vi "Choose_best_target(multi).vi"(0 "R1mag lower limit":dbl, 2 "FOV":dbl, 3 "Footprint":dbl, 5 "PM limit":dbl, 6 "EPOCH TEL":dbl format="%.3f", 8 "DEC TEL":dbl format="%<%H:%M:%S>t", 9 "Table Astrometry":T1 {"CRVAL" format="%.6g"; "CD" format="%_8g"; "NAXIS" format="%#.0f"}, 10 "RA TEL":dbl format="%<%H:%M:%S%1u>t", 12 "USNO_data":string[][](array[string])) -> (11 "Best Target":string[][](array[string]), 13 "erreur":bool, 14 "target RA":dbl format="%<%H:%M:%S%2u>t", 15 "target DEC":dbl format="%<%H:%M:%S%1u>t", 16 "target EPOCH":dbl format="%.3f", 17 "target R1mag":dbl format="%.2f", 18 "target RA (deg)":dbl format="%#.6f", 19 "target DEC (deg)":dbl format="%#.6f")   [LabVIEW 2019]
panel:
  out "tmp_data":string[][](array[string])
  out "R-I":dbl
  out "B-R":dbl
  out "target X":dbl
  out "target Y":dbl
  out "Data OUT":string[][](array[string])
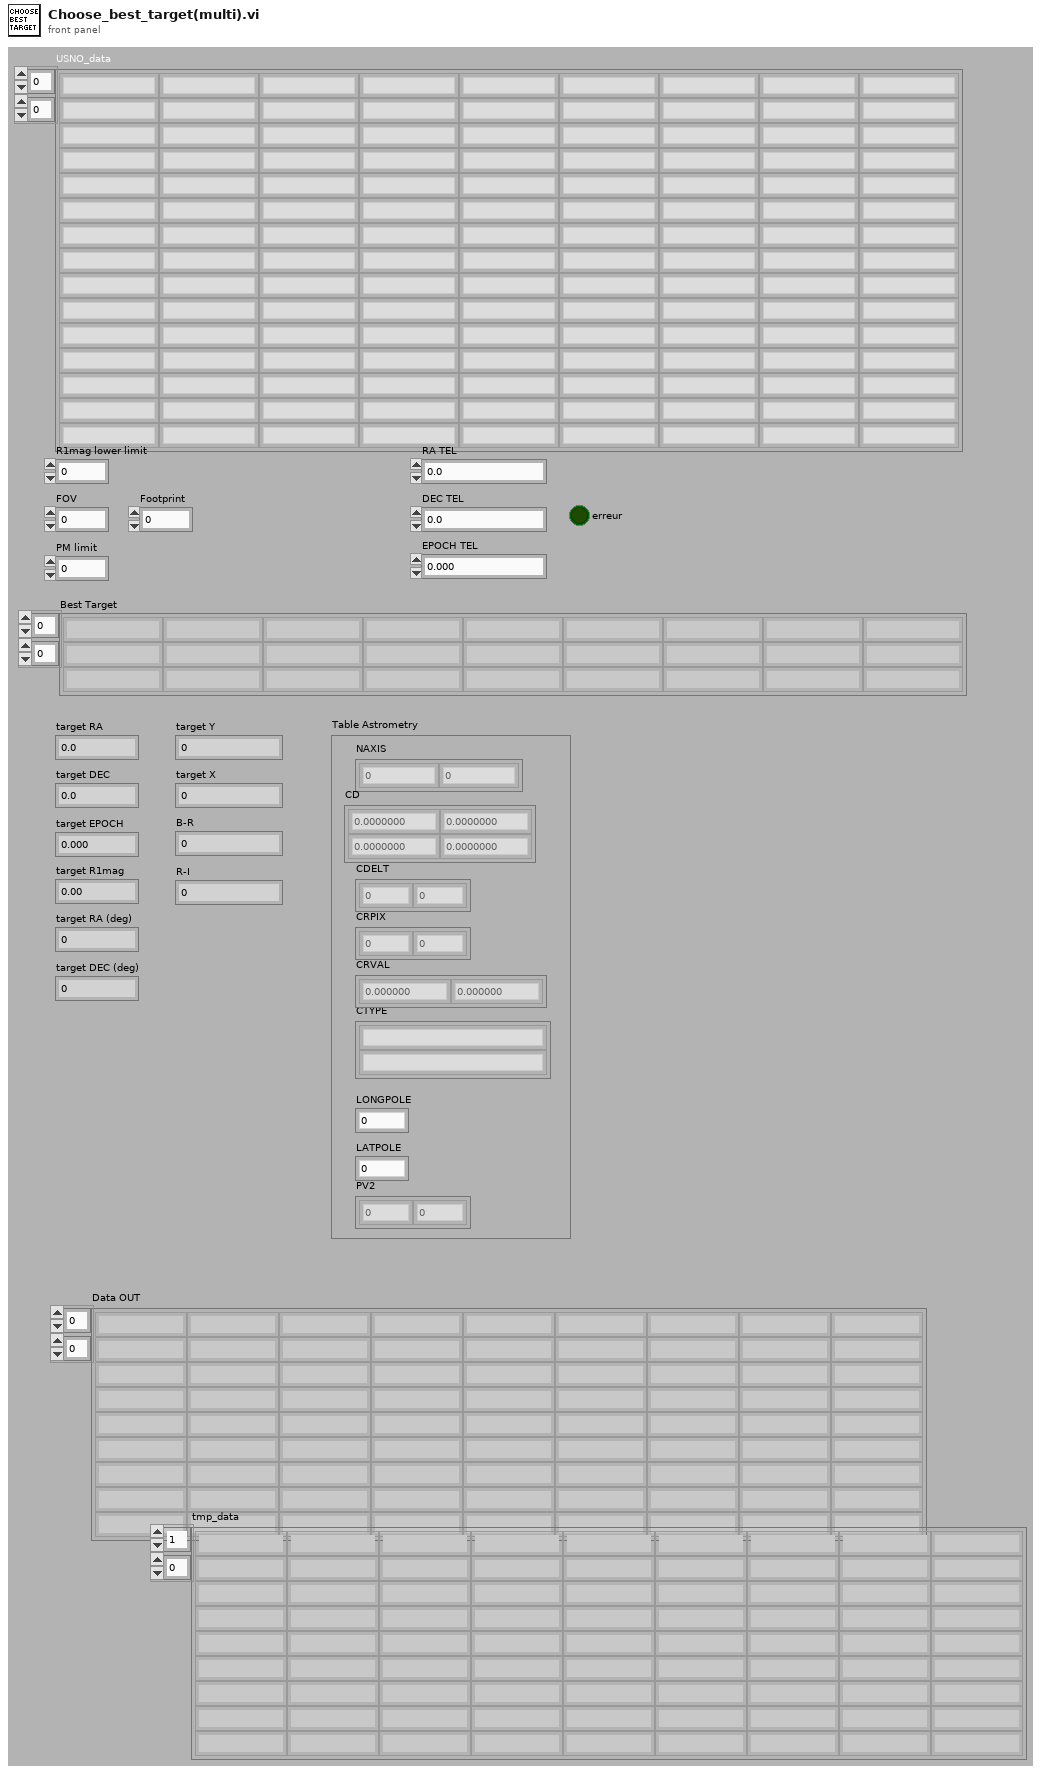
[diagram p1: front panel]
types:
  T1 = cluster{"NAXIS":dbl[], "CD":dbl[][], "CDELT":dbl[], "CRPIX":dbl[], "CTYPE":string[], "CRVAL":dbl[], "LONGPOLE":dbl, "LATPOLE":dbl, "PV2":dbl[]}
  T2 = cluster{"crit":string, "String":string, "String":string, "String":string, "String":string, "String":string, "String":string, "String":string, "String":string}[]
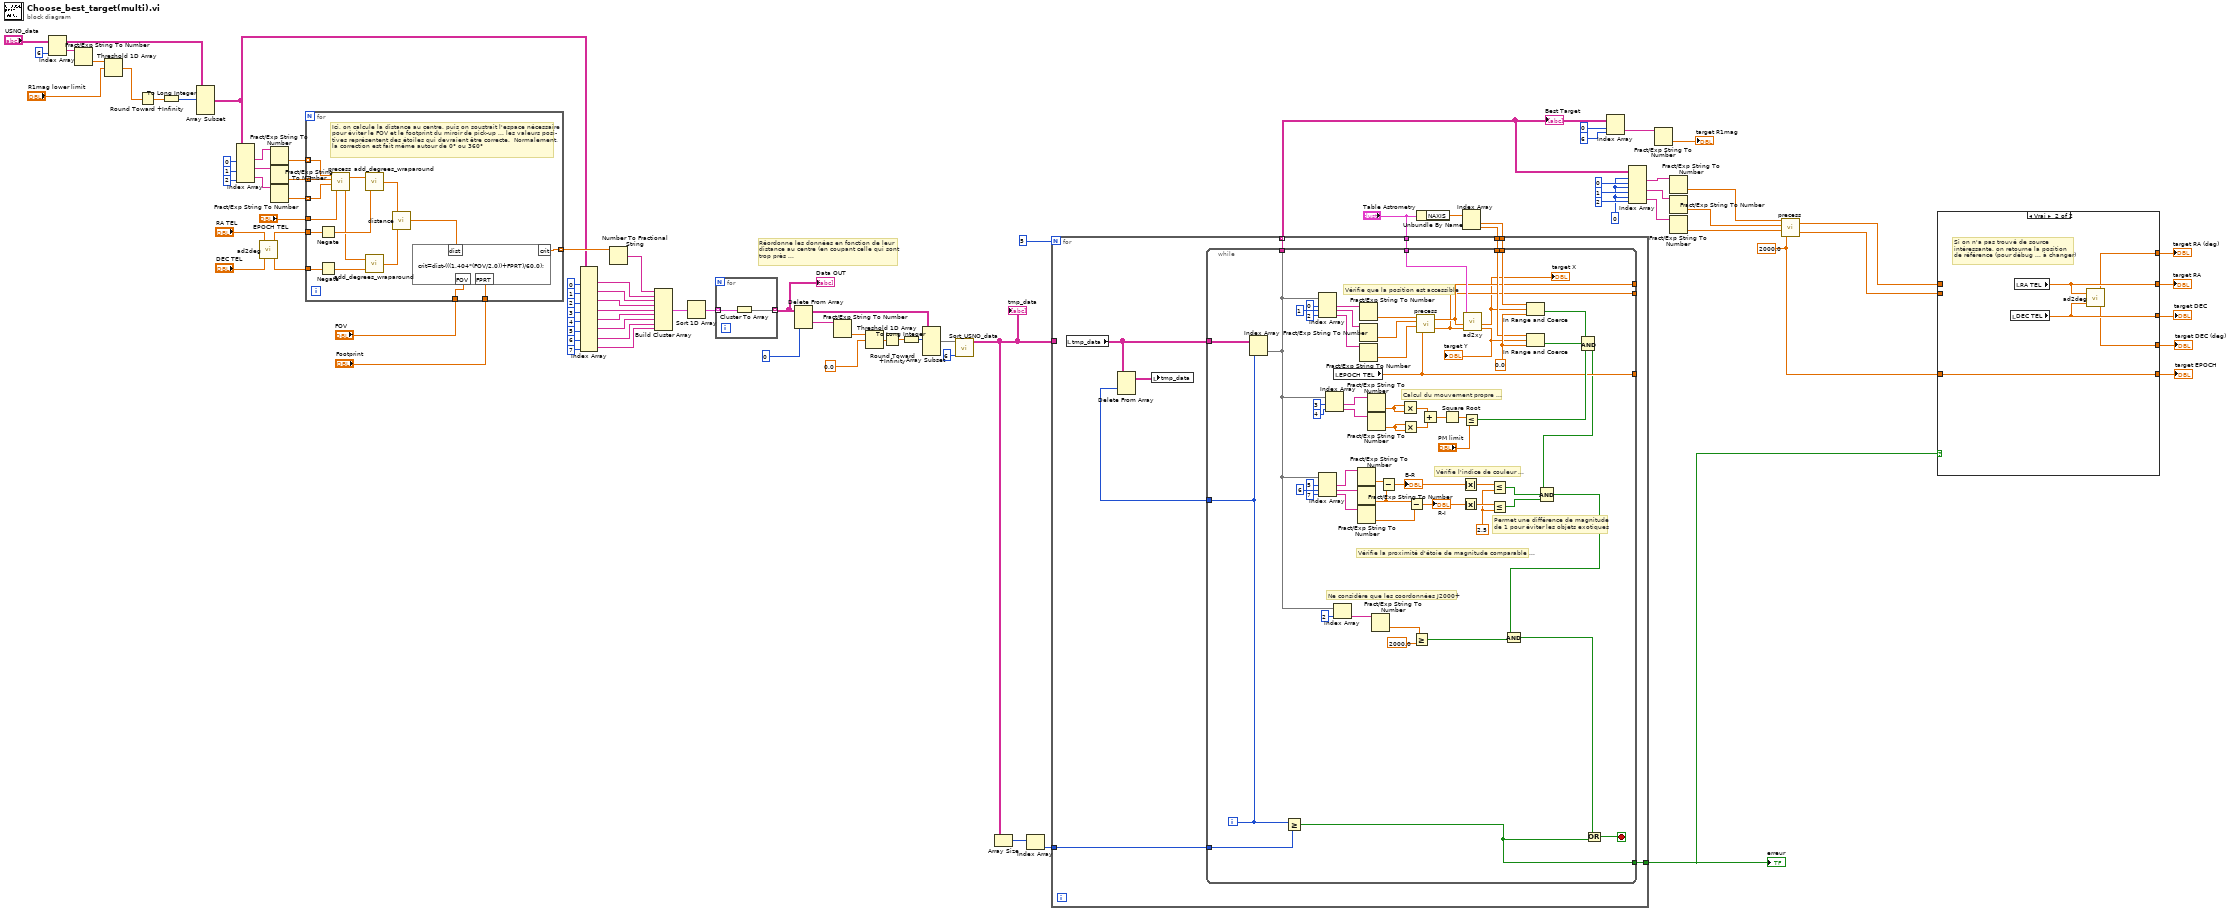
[diagram p0: block diagram]
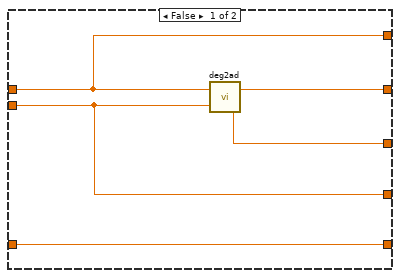
[diagram p2: hidden frame]
diagram:
  w1 = 2000.0 ("Eq2")
  w7 = 0 ("index")
  # "Réordonne les données en fonction de leur\ndistance au centre (en coupant celle qui sont\ntrop près ..."
  n1 = Index Array(array="USNO_data", index (col)=6 ("disabled index (col)")) -> (element=w87:string[])  [unwired: 1 in]
  n2 = Fract/Exp String To Number(string=w87) -> (number=w86:dbl[])  [unwired: 3 in, 1 out]
  n3 = Threshold 1D Array(2:"R1mag lower limit", 3:w86) -> (0:w84:dbl)  [unwired: 1 in]
  n4 = Round Toward +Infinity(x=w84) -> (ceil(x): smallest int >= x=w83:dbl)
  n5 = To Long Integer(number=w83) -> (32bit integer=w82:i32)
  n6 = Array Subset(array="USNO_data", index (row)=w82) -> (w46:string[][])  [unwired: 3 in]
  n7 = Index Array(array=w46, index (col) #1=0 ("disabled index (col)"), index (col) #2=1 ("index (col)"), index (col) #3=2 ("index (col)")) -> (element #1=w78:string[], element #2=w77:string[], element #3=w76:string[])  [unwired: 3 in]
  n8 = call "ad2deg.vi"("DEC (sec)"="DEC TEL", "RA (sec)"="RA TEL") -> ("DEC (°)"=w68:dbl, "RA (°)"=w70:dbl)
  n9 = Fract/Exp String To Number(string=w78) -> (number=w75:dbl[])  [unwired: 3 in, 1 out]
  n10 = Fract/Exp String To Number(string=w77) -> (number=w74:dbl[])  [unwired: 3 in, 1 out]
  n11 = Fract/Exp String To Number(string=w76) -> (number=w73:dbl[])  [unwired: 3 in, 1 out]
  n12 = for {
    tunnel: w75 -> [w104] mode=indexing
    tunnel: w74 -> [w103] mode=indexing
    tunnel: w73 -> [w102] mode=indexing
    tunnel: "EPOCH TEL" -> [w101]
    tunnel: w70 -> [w100]
    tunnel: w68 -> [w99]
    tunnel: "FOV" -> [w91]
    tunnel: "Footprint" -> [w92]
    tunnel: [w89] -> w47 mode=indexing
    # "Ici, on calcule la distance au centre, puis on soustrait l'espace nécessaire\npour éviter le FOV et le footprint du miroir de pick-up ... les valeurs posi-\ntives représentent des étoiles qui devraient être correcte.  Normalement,\nla correction est fait même autour de 0° ou 360°"
    n13 = Negate(x=w100) -> (-x=w97:dbl)
    n14 = Negate(x=w99) -> (-x=w96:dbl)
    n15 = call "precess.vi"("Eq2"=w101, "Eq1"=w102, "DEC 1"=w103, "RA 1"=w104) -> ("DEC 2"=w95:dbl, "RA 2"=w98:dbl)
    n16 = call "add_degrees_wraparound.vi"("DEG 2"=w97, "DEG 1"=w98) -> ("DEG OUT"=w94:dbl)
    n17 = call "add_degrees_wraparound.vi"("DEG 2"=w96, "DEG 1"=w95) -> ("DEG OUT"=w93:dbl)
    n18 = call "distance.vi"("D2"=w93, "D1"=w94) -> ("DT"=w90:dbl)
    n19 = formula code="crit=dist-(((1.404*(FOV/2.0))+FPRT)/60.0);"("FOV"=w91, "FPRT"=w92, "dist"=w90) -> ("crit"=w89:dbl)
  }
  n20 = Index Array(array=w46, index (col) #1=0 ("index (col)"), index (col) #2=1 ("index (col)"), index (col) #3=2 ("index (col)"), index (col) #4=3 ("index (col)"), index (col) #5=4 ("index (col)"), index (col) #6=5 ("index (col)"), index (col) #7=6 ("index (col)"), index (col) #8=7 ("index (col)")) -> (element #1=w56:string[], element #2=w57:string[], element #3=w58:string[], element #4=w59:string[], element #5=w60:string[], element #6=w61:string[], element #7=w62:string[], element #8=w63:string[])  [unwired: 8 in]
  n21 = Number To Fractional String(number=w47) -> (F-format string=w45:string[])  [unwired: 3 in]
  n22 = Build Cluster Array(w45, w56, w57, w58, w59, w60, w61, w62, w63) -> (w64:T2)
  n23 = Sort 1D Array(array=w64) -> (sorted array=w65:T2)
  n24 = for {
    tunnel: w65 -> [w106] mode=indexing
    tunnel: [w105] -> w26 mode=indexing
    n25 = Cluster To Array(cluster=w106) -> (array=w105:string[])
  }
  "Data OUT" <- w26
  n26 = Delete From Array(array=w26, index (col)=0 ("disabled index (col)")) -> (deleted portion=w44:string[], array with subset deleted=w35:string[][])  [unwired: 2 in]
  n27 = Fract/Exp String To Number(string=w44) -> (number=w43:dbl[])  [unwired: 3 in, 1 out]
  n28 = Threshold 1D Array(2:0.0 ("threshold y"), 3:w43) -> (0:w39:dbl)  [unwired: 1 in]
  n29 = Round Toward +Infinity(x=w39) -> (ceil(x): smallest int >= x=w40:dbl)
  n30 = To Long Integer(number=w40) -> (32bit integer=w41:i32)
  n31 = Array Subset(array=w35, index (row)=w41) -> (w38:string[][])  [unwired: 3 in]
  n32 = call "Sort_USNO_data.vi"("Column Used"=6, "Data IN"=w38) -> ("Data OUT"=w25:string[][])  [unwired: 8 in, 1 out]
  "tmp_data" <- w25
  n33 = Array Size(array=w25) -> (size(s)=w27:i32[])
  n34 = Index Array(array=w27) -> (element=w24:i32)  [unwired: 1 in]
  n35 = Unbundle By Name("Table Astrometry") -> ("NAXIS"=w34:dbl[])
  n36 = Index Array(array=w34) -> (element #1=w32:dbl, element #2=w31:dbl)  [unwired: 2 in]
  n37 = for {
    N: 5 -> [_]
    tunnel: "Table Astrometry" -> [w115]
    tunnel: w32 -> [w114]
    tunnel: w31 -> [w113]
    tunnel: [w112] -> w11 mode=indexing
    tunnel: w25 -> [_]
    tunnel: w24 -> [w111]
    tunnel: [w110] -> w23
    n38 = local read "tmp_data"() -> (w109:string[][])
    n39 = while {
      tunnel: w109 -> [w125]
      tunnel: w115 -> [w157]
      tunnel: w114 -> [w155]
      tunnel: w113 -> [w154]
      tunnel: [w150] -> _
      tunnel: [w149] -> _
      tunnel: [w148] -> _
      tunnel: [w123] -> w112
      tunnel: w111 -> [w144]
      tunnel: [w143] -> w110
      tunnel: [w124] -> w107
      i -> [w124]
      stop <- w145 stop-if-true
      w129 = 2.5 ("y")
      w156 = 0.0
      # "Ne considère que les coordonnées J2000+"
      # "Vérifie la proximité d'étoie de magnitude comparable ..."
      # "Permet une différence de magnitude\nde 1 pour éviter les objets exotiques"
      # "Vérifie l'indice de couleur ..."
      # "Vérifie que la position est accessible"
      # "Calcul du mouvement propre ..."
      n40 = Index Array(array=w125, index (row)=w124) -> (element=w123:string[])  [unwired: 1 in]
      n41 = Greater Or Equal?(x=w124, y=w144) -> (x >= y?=w143:bool)
      n42 = Index Array(array=w123, index #1=0 ("index"), index #2=1 ("index"), index #3=2 ("index")) -> (element #1=w161:string, element #2=w160:string, element #3=w163:string)
      n43 = Index Array(array=w123, index #1=5 ("index (row)"), index #2=6 ("index (row)"), index #3=7 ("index")) -> (element #1=w139:string, element #2=w138:string, element #3=w137:string)
      n44 = Index Array(array=w123, index #1=3 ("index (row)"), index #2=4 ("index (row)")) -> (element #1=w171:string, element #2=w172:string)
      n45 = local read "EPOCH TEL"() -> (w148:dbl)
      n46 = Index Array(array=w123, index=2) -> (element=w121:string)
      n47 = Fract/Exp String To Number(string=w139) -> (number=w136:dbl)  [unwired: 3 in, 1 out]
      n48 = Fract/Exp String To Number(string=w138) -> (number=w135:dbl)  [unwired: 3 in, 1 out]
      n49 = Fract/Exp String To Number(string=w137) -> (number=w134:dbl)  [unwired: 3 in, 1 out]
      n50 = Fract/Exp String To Number(string=w161) -> (number=w166:dbl)  [unwired: 3 in, 1 out]
      n51 = Fract/Exp String To Number(string=w160) -> (number=w165:dbl)  [unwired: 3 in, 1 out]
      n52 = Fract/Exp String To Number(string=w163) -> (number=w164:dbl)  [unwired: 3 in, 1 out]
      n53 = Fract/Exp String To Number(string=w171) -> (number=w173:dbl)  [unwired: 3 in, 1 out]
      n54 = Fract/Exp String To Number(string=w172) -> (number=w174:dbl)  [unwired: 3 in, 1 out]
      n55 = Fract/Exp String To Number(string=w121) -> (number=w120:dbl)  [unwired: 3 in, 1 out]
      n56 = Subtract(x=w136, y=w135) -> (x-y=w133:dbl)
      "B-R" <- w133
      n57 = Multiply(x=w173, y=w173) -> (x*y=w175:dbl)
      n58 = Multiply(x=w174, y=w174) -> (x*y=w176:dbl)
      n59 = Subtract(x=w135, y=w134) -> (x-y=w132:dbl)
      "R-I" <- w132
      n60 = Greater Or Equal?(x=w120, y=2000.0) -> (x >= y?=w117:bool)
      n61 = call "precess.vi"("Eq2"=w148, "Eq1"=w164, "DEC 1"=w165, "RA 1"=w166) -> ("DEC 2"=w149:dbl, "RA 2"=w150:dbl)
      n62 = Add(x=w175, y=w176) -> (x+y=w177:dbl)
      n63 = Square Root(x=w177) -> (sqrt(x)=w168:dbl)
      n64 = Absolute Value(x=w133) -> (abs(x)=w131:dbl)
      n65 = Absolute Value(x=w132) -> (abs(x)=w130:dbl)
      n66 = Less Or Equal?(x=w168, y="PM limit") -> (x <= y?=w153:bool)
      n67 = call "ad2xy.vi"("DEC"=w149, "RA"=w150, "Astrometry"=w157) -> ("Y"=w146:dbl, "X"=w147:dbl)  [unwired: 6 in, 1 out]
      "target Y" <- w146
      "target X" <- w147
      n68 = Less Or Equal?(x=w131, y=w129) -> (x <= y?=w128:bool)
      n69 = Less Or Equal?(x=w130, y=w129) -> (x <= y?=w127:bool)
      n70 = In Range and Coerce(upper limit=w155, x=w147, lower limit=w156) -> (In Range?=w152:bool)  [unwired: 1 out]
      n71 = In Range and Coerce(upper limit=w154, x=w146, lower limit=w156) -> (In Range?=w151:bool)  [unwired: 1 out]
      n72 = Compound Arithmetic op=AND(w152, w151, w153) -> (w126:bool)
      n73 = Compound Arithmetic op=AND(w126, w128, w127) -> (w118:bool)
      n74 = Compound Arithmetic op=AND(w118, w117) -> (w116:bool)
      n75 = Or(x=w116, y=w143) -> (x .or. y?=w145:bool)
    }
    n76 = Delete From Array(array=w109, index (row)=w107) -> (array with subset deleted=w108:string[][])  [unwired: 2 in, 1 out]
    n77 = local write "tmp_data"(w108) -> ()
  }
  "Best Target" <- w11
  "erreur" <- w23
  n78 = Index Array(array=w11, index (row)=0 ("index"), index (col)=6 ("disabled index (col)")) -> (element=w29:string)
  n79 = Index Array(array=w11, index (row) #1=w7, index (col) #1=0 ("index"), index (row) #2=w7, index (col) #2=1 ("index"), index (row) #3=w7, index (col) #3=2 ("index")) -> (element #1=w13:string, element #2=w14:string, element #3=w12:string)
  n80 = Fract/Exp String To Number(string=w29) -> (number=→"target R1mag":dbl)  [unwired: 3 in, 1 out]
  n81 = Fract/Exp String To Number(string=w13) -> (number=w6:dbl)  [unwired: 3 in, 1 out]
  n82 = Fract/Exp String To Number(string=w14) -> (number=w5:dbl)  [unwired: 3 in, 1 out]
  n83 = Fract/Exp String To Number(string=w12) -> (number=w4:dbl)  [unwired: 3 in, 1 out]
  n84 = call "precess.vi"("Eq2"=w1, "Eq1"=w4, "DEC 1"=w5, "RA 1"=w6) -> ("DEC 2"=w2:dbl, "RA 2"=w3:dbl)
  n85 = case shown="Vrai" w23 {
    tunnel: w1 -> [w178 w183]
    tunnel: w3 -> [w179 _]
    tunnel: w2 -> [w180 _]
    tunnel: [w182 w186] -> w19
    tunnel: [w181 w187] -> w18
    tunnel: [w180 w184] -> w17
    tunnel: [w179 w185] -> w16
    tunnel: [w178 w183] -> w15
    frame False {
      n86 = call "deg2ad.vi"("DEC (°)"=w180, "RA (°)"=w179) -> ("DEC (°)"=w181:dbl, "RA (sec)"=w182:dbl)
    }
    frame True {
      # "Si on n'a pas trouvé de source\nintéressante, on retourne la position\nde référence (pour débug ... à changer)"
      n87 = local read "DEC TEL"() -> (w187:dbl)
      n88 = local read "RA TEL"() -> (w186:dbl)
      n89 = call "ad2deg.vi"("DEC (sec)"=w187, "RA (sec)"=w186) -> ("DEC (°)"=w184:dbl, "RA (°)"=w185:dbl)
    }
  }
  "target RA" <- w19
  "target DEC" <- w18
  "target DEC (deg)" <- w17
  "target RA (deg)" <- w16
  "target EPOCH" <- w15
